vi "Sampler.vi"(5 "Meas. Time (1 s) (0.01 - 10)":dbl=1.0, 7 "Loops (10) (1 - 1000)":i32=10, 8 "error in (no error)":errorcluster, 9 "Trigger Slope (F)":bool, 10 "Result as Mean? (F)":bool, 11 "Vertical Range (V)":dbl=5.0) -> (0 "error out":errorcluster, 2 "RMS Voltages (V)":dbl[](array[numeric]) format="%#_9g", 4 "Std. Dev. (V)":dbl, 6 "Mean (V)":dbl)   [LabVIEW 2019, in "ACSVcontrol-driver.lvlib"]
doc: "Returns readings from the nulldetector. This VI is not finished and is missing some possibilities.\n\nThe PJVS.vi (command “Set_PJVS”) with an AC waveform must be used before read out the sampler, otherwise Trigger and Clock will not be set for PXI and Waveform Generator.\n\nIf \"Trigger Slope\" is True, the read out of the Sampler starts with the rising edge of the trigger signal. Vertical Range is coerced to 1 V pp or 5 V pp. Loops is the number of measurements. The number of periods to be measured will be calculated by the supraVOLTcontrol software.\n\nIf \"Result as Mean\" is True, output of the VI is mean and standard deviation, otherwise all RMS values are returned.\n If Loops = 1 and Result as Mean is False, result is samples of PXI for one period without transients and all periods are averaged to one period.\n\nIf the multiplexer is set to \"Short Switch AC\", also Gain & Offset of PXI is returned. These va6lues will be updated in the supraVOLTcontrol software only in case the measured value for gain is in range between 0.999 to 1.001. For the next Measurement the new gain and offset will be taken into account."
uses:
  ACSVcontrol-driver.lvlib
  Private/Type definitions/Command.ctl
  Private/Type definitions/Status.ctl
  Private/Type definitions/Instruction.ctl
  Private/Globals.vi
  <vilib>/Utility/error.llb/Error Cluster From Error Code.vi
  <vilib>/ErrorRing/Error Ring.xnode
  <vilib>/Analysis/NI_AALBase.lvlib
panel:
  out "resulting string":string
  in  "number format string":string="%.6f"
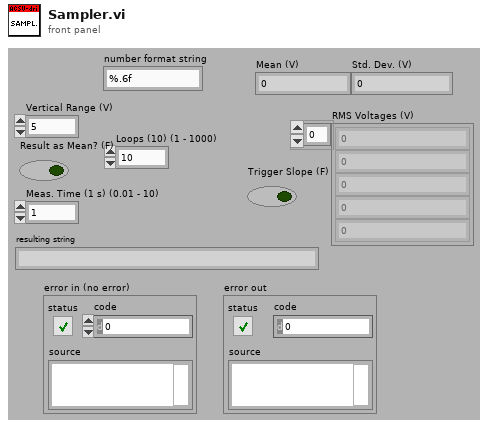
[diagram p1: front panel]
types:
  T1 = typedef "ACSVcontrol-driver.lvlib/Status.ctl" = enum16{"waiting", "processing", "error command", "Set_PJVS-Done", "Set_Mux-Done", "Set_Mux-Error", "Set_57XX-Done", "Set_57XX-Error", "Set_Gen-Done", "Set_Gen-Error", "Set_Synthesizer-Done", "Set_Synthesizer-Error", "Read_Nano-Done", "Read_Sampler-Done", "Read_Sampler-Error", "Read_Sensors-Done"}
  T2 = typedef "ACSVcontrol-driver.lvlib/Command.ctl" = enum16{"Set_PJVS", "Set_Mux", "Set_57XX", "Set_Gen", "Set_Synthesizer", "Read_Nulldetector", "Read_Sampler", "Read_Sensors"}
  T3 = typedef "ACSVcontrol-driver.lvlib/Instruction.ctl" = enum16{"dummy - do not use", "Send Command", "Read Result", "Ask Status"}
  T4 = typedef "ACSVcontrol-driver.lvlib/Timeouts.ctl" = cluster{"TCP Read & Write (ms)":i32, "Sensors readout":i32, "PJVS setup":i32, "Nullmeter readout":i32, "Multiplexer setup":i32, "57XX setup":i32, "Generator setup":i32, "Synthesizer setup":i32, "Sampler readout":i32}
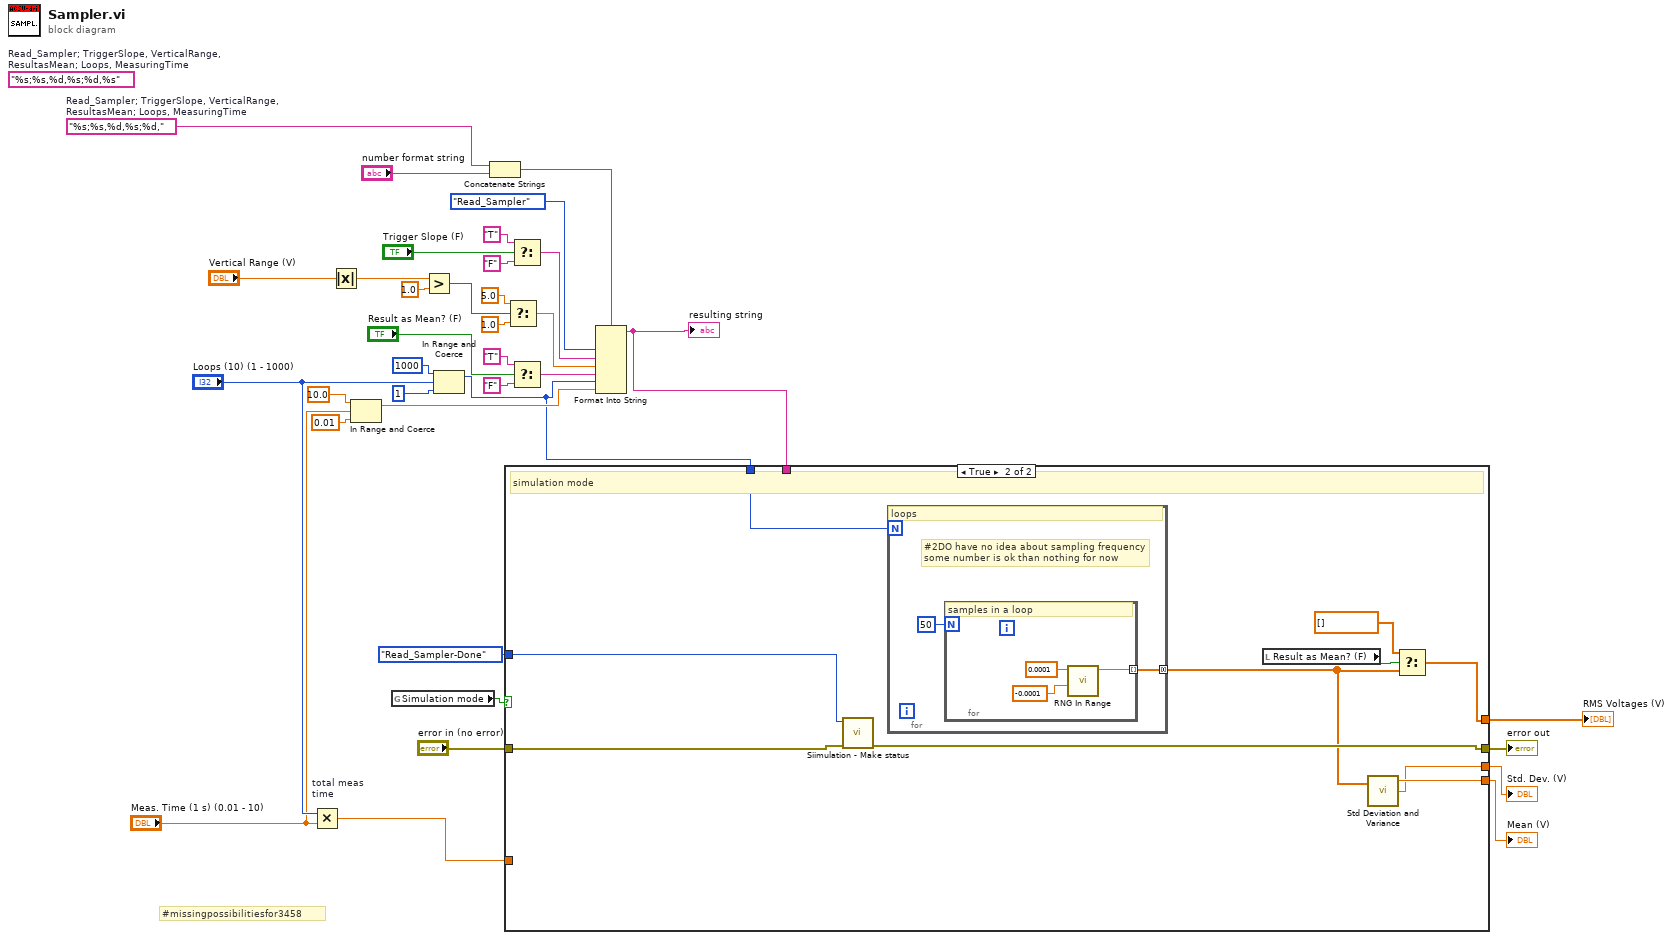
[diagram p0: block diagram]
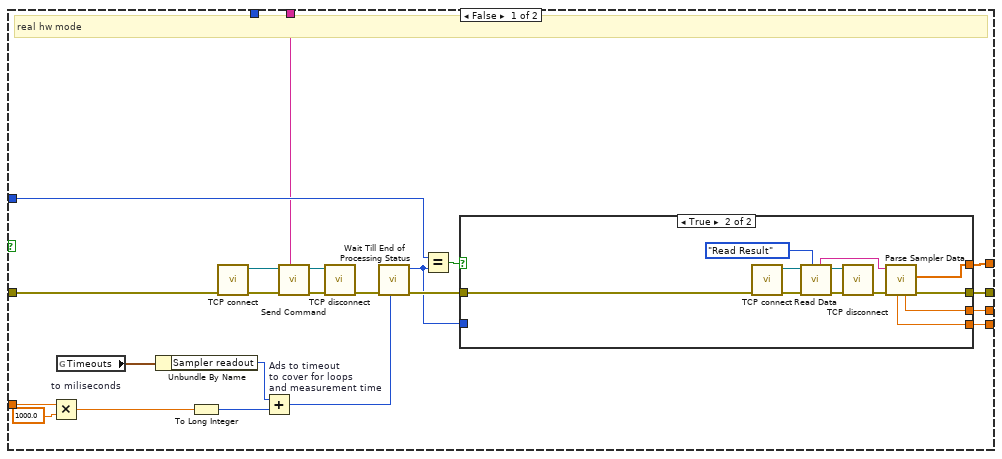
[diagram p2: hidden frame]
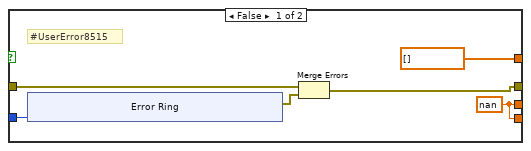
[diagram p3: hidden frame]
diagram:
  w10 = "%s;%s,%d,%s;%d,"  # Read_Sampler; TriggerSlope, VerticalRange, ResultasMean; Loops, MeasuringTime
  (unwired) "%s;%s,%d,%s;%d,%s"  # Read_Sampler; TriggerSlope, VerticalRange, ResultasMean; Loops, MeasuringTime
  # "#missingpossibilitiesfor3458"
  n1 = Multiply "total meas\ntime"(x="Loops (10) (1 - 1000)", y="Meas. Time (1 s) (0.01 - 10)") -> (x*y=w5:dbl)
  n2 = Absolute Value(x="Vertical Range (V)") -> (abs(x)=w21:dbl)
  n3 = In Range and Coerce(upper limit=10.0 ("x"), x="Meas. Time (1 s) (0.01 - 10)", lower limit=0.01 ("x")) -> (coerced(x)=w8:dbl)  [unwired: 1 out]
  n4 = global read "Globals.vi" "Simulation mode"() -> (w2:bool)
  n5 = Greater?(x=w21, y=1.0 ("x")) -> (0:w22:bool)
  n6 = In Range and Coerce(upper limit=1000, x="Loops (10) (1 - 1000)", lower limit=1) -> (coerced(x)=w1:i32)  [unwired: 1 out]
  n7 = Concatenate Strings(w10, "number format string") -> (w9:string)
  n8 = Select(t=5.0 ("y"), s=w22, f=1.0) -> (s? t:f=w18:dbl)
  n9 = Select(t="T" ("format string"), s="Trigger Slope (F)", f="F" ("format string")) -> (s? t:f=w25:string)
  n10 = Select(t="T" ("format string"), s="Result as Mean? (F)", f="F" ("format string")) -> (s? t:f=w14:string)
  n11 = Format Into String(format string=w9, Command."Read_Sampler" ("Command"), w25, w18, w14, w1, w8) -> (resulting string=w29:string)  [unwired: 2 in, 1 out]
  "resulting string" <- w29
  n12 = case shown="True" w2 {
    tunnel: "error in (no error)" -> [w58 w93]
    tunnel: Status."Read_Sampler-Done" ("x") -> [w52 w91]
    tunnel: [w48 w92] -> w31
    tunnel: [w47 w86] -> w30
    tunnel: w29 -> [w45 _]
    tunnel: [w44 w89] -> w7
    tunnel: [w43 w88] -> w6
    tunnel: w5 -> [w39 _]
    tunnel: w1 -> [_ w90]
    frame False {
      # "real hw mode"
      n13 = Multiply "to miliseconds"(x=w39, y=1000.0) -> (x*y=w41:dbl)
      n14 = global read "Globals.vi" "Timeouts"() -> (w46:T4)
      n15 = Unbundle By Name(w46) -> ("Sampler readout"=w38:i32)
      n16 = To Long Integer(number=w41) -> (32bit integer=w42:i32)
      n17 = call "TCP connect.vi"("error in (no error)"=w58) -> ("error out"=w57:errorcluster, "connection ID"=w56:refnum<k5>)  [unwired: 9 in]
      n18 = Add "Ads to timeout\nto cover for loops\nand measurement time"(x=w38, y=w42) -> (x+y=w37:i32)
      n19 = call "Send Command.vi"("Command"=w45, "error in (no error)"=w57, "connection ID"=w56) -> ("error out"=w55:errorcluster, "connection ID out"=w54:refnum<k5>)  [unwired: 7 in]
      n20 = call "TCP disconnect.vi"("error in (no error)"=w55, "connection ID"=w54) -> ("error out"=w49:errorcluster)  [unwired: 9 in]
      n21 = call "Wait Till End of Processing Status.vi"("Loop Timeout (ms) (5000)"=w37, "error in (no error)"=w49) -> ("error out"=w53:errorcluster, "Last Status"=w50:T1)  [unwired: 8 in]
      n22 = Equal?(x=w52, y=w50) -> (x = y?=w51:bool)
      n23 = case shown="True" w51 {
        tunnel: w53 -> [w64 w81]
        tunnel: [w61 w76] -> w48
        tunnel: w50 -> [w63 _]
        tunnel: [dbl[] [] ("Relative times (s)") w75] -> w47
        tunnel: [w59 w73] -> w44
        tunnel: [w59 w72] -> w43
        frame False {
          w59 = nan
          # "#UserError8515"
          n24 = xnode "Error Ring"("parameter 0"=w63) -> ("error out"=w62:errorcluster)
          n25 = Merge Errors(w64, w62) -> (w61:errorcluster)
        }
        frame True {
          n26 = call "TCP connect.vi"("error in (no error)"=w81) -> ("error out"=w80:errorcluster, "connection ID"=w79:refnum<k5>)  [unwired: 9 in]
          n27 = call "Read Data.vi"("Instruction"=Instruction."Read Result", "error in (no error)"=w80, "connection ID"=w79) -> ("error out"=w83:errorcluster, "connection ID out"=w82:refnum<k5>, "Data"=w74:string)  [unwired: 6 in]
          n28 = call "TCP disconnect.vi"("error in (no error)"=w83, "connection ID"=w82) -> ("error out"=w77:errorcluster)  [unwired: 9 in]
          n29 = call "Parse Sampler Data.vi"("error in"=w77, "Data"=w74) -> ("error out"=w76:errorcluster, "Voltages (V)"=w75:dbl[], "Std. Dev. (V)"=w72:dbl, "Mean (V)"=w73:dbl)  [unwired: 6 in]
        }
      }
    }
    frame True {
      # "simulation mode"
      n30 = call "Siimulation - Make status.vi"("error in (no error)"=w93, "Status"=w91) -> ("error out"=w92:errorcluster)  [unwired: 8 in, 1 out]
      n31 = for {
        N: w90 -> [_]
        tunnel: [w95] -> w87 mode=concatenating
        # "#2DO have no idea about sampling frequency\nsome number is ok than nothing for now"
        # "loops"
        n32 = for {
          N: 50 -> [_]
          tunnel: [w98] -> w95 mode=indexing
          # "samples in a loop"
          n33 = call "RNG In Range.vi"("llimit 2 (1)"=-0.0001 ("upper bound (100)"), "limit 1 (0)"=0.0001 ("upper bound (100)")) -> ("number"=w98:dbl)  [unwired: 9 in]
        }
      }
      n34 = local read "Result as Mean? (F)"() -> (w84:bool)
      n35 = call <vilib>:"Std Deviation and Variance.vi"("X"=w87) -> ("mean"=w89:dbl, "standard deviation"=w88:dbl)  [unwired: 1 in, 1 out]
      n36 = Select(t=dbl[] [] ("array type (2D Dbl)"), s=w84, f=w87) -> (s? t:f=w86:dbl[])
    }
  }
  "error out" <- w31
  "RMS Voltages (V)" <- w30
  "Mean (V)" <- w7
  "Std. Dev. (V)" <- w6
